vi "SetOscillatorPan.vi"(8 "error in (no error)":errorcluster caption="entrée d'erreur (pas d'erreur)", 11 "EGG5210.lvclass":refnum<class "EGG5210.lvclass">) -> (0 "error out":errorcluster caption="sortie d'erreur", 3 "EGG5210.lvclass Out":refnum<class "EGG5210.lvclass">)   [LabVIEW 2010, in "EGG5210.lvclass"]
uses:
  EGG5210.lvclass
  BaseDevice/BaseDevice.lvclass
panel:
  in  "Acq":bool
  in  "Amplitude":dbl
  in  "Frequency":dbl
  in  "Stop":bool
  in  "MiseAJour":bool
  out "Init Program":bool
  # "EG&G 5210\nOscillator"
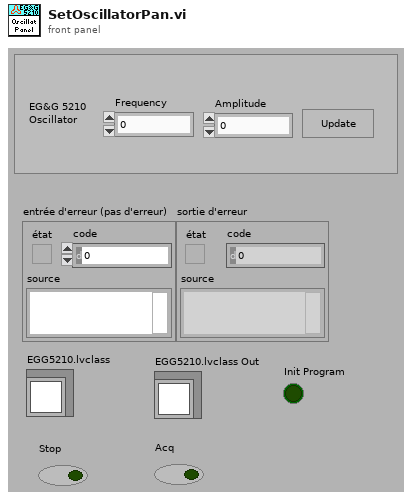
[diagram p1: front panel]
types:
  T1 = enum8{"Enabled", "Disabled", "Disabled and Grayed Out"}
  T2 = enum16{"X Output", "Y Output", "X and Y Output", "Mag", "Phase", "Mag & Phase", "X,Y,Mag & Phase", "Noise", "Aux In 1", "Aux In 2", "Aux In 3", "Aux In 4"}
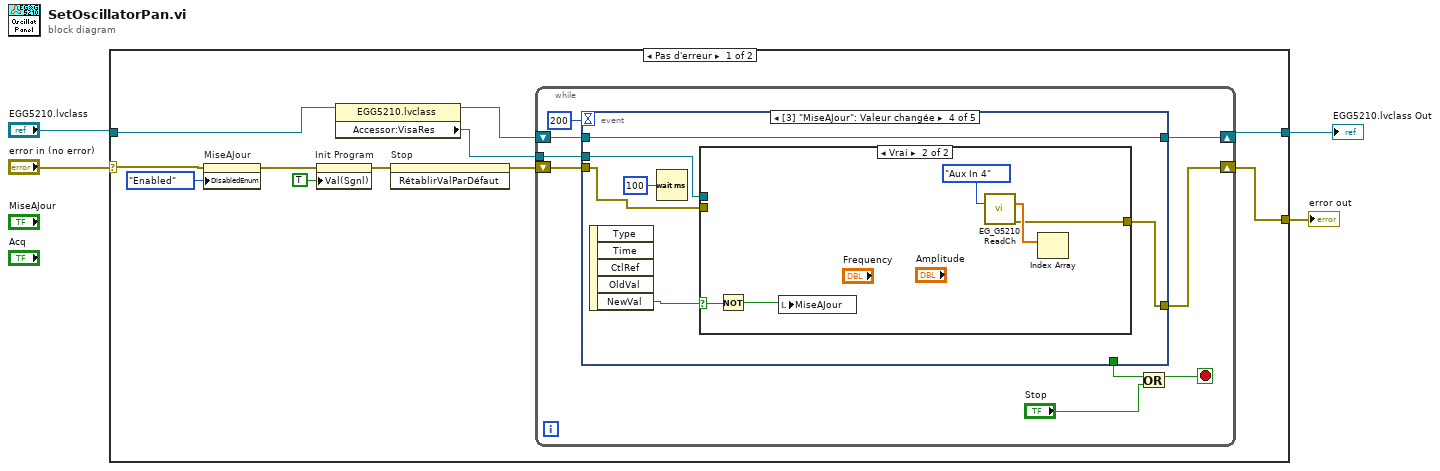
[diagram p0: block diagram]
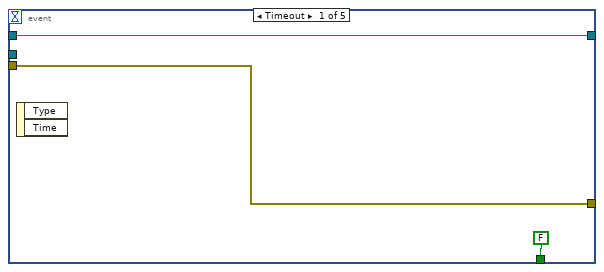
[diagram p2: hidden frame]
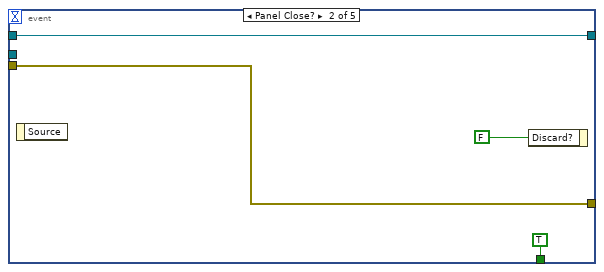
[diagram p3: hidden frame]
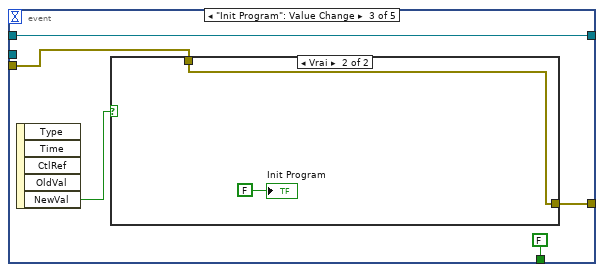
[diagram p4: hidden frame]
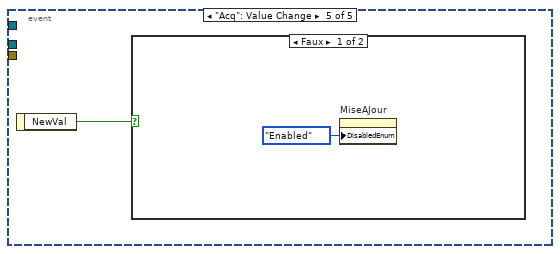
[diagram p7: hidden frame]
diagram:
  n1 = case shown="Pas d'erreur" "error in (no error)" {
    selector: "error in (no error)" -> [w6 w57]
    tunnel: [w15 w57] -> w3
    tunnel: "EGG5210.lvclass" -> [w10 w56]
    tunnel: [w13 w56] -> w2
    frame No Error {
      n2 = property on="MiseAJour" class="Bool (strict)"(error in=w6, "DisabledEnum"=T1."Enabled" ("Désactivé")) -> (error out=w5:errorcluster)  [unwired: 1 in, 1 out]
      n3 = property on="Init Program" class="Bool (strict)"(error in=w5, "Val(Sgnl)"=TRUE ("Valeur (Signalisation)")) -> (error out=w12:errorcluster)  [unwired: 1 in, 1 out]
      n4 = property class="EGG5210.lvclass"(reference=w10) -> (reference out=w9:refnum<class "EGG5210.lvclass">, "Accessor:VisaRes"=w8:refnum<visa-resource-name>)  [unwired: 1 in, 1 out]
      n5 = invoke on="Stop" class="Bool (strict)" method="RétablirValParDéfaut"(error in=w12) -> (error out=w11:errorcluster)  [unwired: 2 in, 2 out]
      n6 = while {
        shift-right: [w22] -> w15
        shift-left: w11 -> [w23]
        shift-right: [w19] -> w13
        shift-left: w9 -> [w21]
        tunnel: w8 -> [w16]
        stop <- w18 stop-if-true
        n7 = event shown="[3] \"MiseAJour\": Valeur changée" {
          selector: _ -> [_ _ _ _ _]
          dyn-events: _ -> [_ _ _ _ _]
          timeout: 200 -> [_ _ _ _ _]
          tunnel: w23 -> [w25 w29 w35 w41 _]
          tunnel: [w25 w29 w34 w40 _] -> w22
          tunnel: w21 -> [w26 w28 w33 w42 _]
          tunnel: [FALSE TRUE FALSE _ _] -> w20
          tunnel: [w26 w28 w33 w42 _] -> w19
          tunnel: w16 -> [_ _ _ w43 _]
          event Timeout {
            n8 = event-data() -> ()  [unwired: 1 in, 2 out]
          }
          event Panel Close? {
            n9 = event-data() -> ()  [unwired: 1 in, 1 out]
            n10 = event-data("Discard?"=FALSE ("Rejeter ?")) -> ()  [unwired: 1 in, 1 out]
          }
          event "Init Program": Value Change {
            n11 = event-data() -> ("NewVal"=w36:bool)  [unwired: 1 in, 4 out]
            n12 = case shown="Vrai" w36 {
              tunnel: w35 -> [w37 w38]
              tunnel: [w37 w38] -> w34
              frame False {
              }
              frame True {
                "Init Program" <- FALSE
              }
            }
          }
          event "MiseAJour": Value Change {
            n13 = event-data() -> ("NewVal"=w44:bool)  [unwired: 1 in, 4 out]
            n14 = Wait (ms)(milliseconds to wait=u32 100 ("attente (ms)")) -> ()  [unwired: 1 out]
            n15 = case shown="Vrai" w44 {
              selector: w44 -> [_ w53]
              tunnel: w43 -> [_ _]
              tunnel: w41 -> [w46 _]
              tunnel: [w46 w47] -> w40
              frame False {
              }
              frame True {
                n16 = Not(x=w53) -> (.not. x?=w52:bool)
                n17 = local write "MiseAJour"(w52) -> ()
                n18 = call <userlib>:"EG_G5210 ReadCh.vi"("Channel"=T2."Aux In 4") -> ("VISA Rsrc"=w49:refnum<visa-resource-name>, "Outputs"=w48:dbl[], "error in (no error)"=w50:errorcluster, "error out"=w47:errorcluster)  [unwired: 5 in, 6 out]
                n19 = Index Array(array=w48) -> ()  [unwired: 1 in, 1 out]
              }
            }
          }
          event "Acq": Value Change {
            n20 = event-data() -> ("NewVal"=w54:bool)  [unwired: 1 in]
            n21 = case shown="Faux" w54 {
              frame False {
                n22 = property on="MiseAJour" class="Bool (strict)"("DisabledEnum"=T1."Enabled" ("Désactivé")) -> ()  [unwired: 2 in, 2 out]
              }
              frame True {
              }
            }
          }
        }
        n23 = Or(x=w20, y="Stop") -> (x .or. y?=w18:bool)
      }
    }
    frame Error {
    }
  }
  "error out" <- w3
  "EGG5210.lvclass Out" <- w2
